vi "OpenPattern.vi"(8 "Error In":errorcluster, 11 "Patten File Path":path caption="path to XML document") -> (0 "Error Out":errorcluster, 3 "Pattern":T1)   [LabVIEW 2012, in "Virtual-PGA.lvlib"]
doc: "This VI loads a pattern from a XML file. The \"Select Pattern Load File Path\" VI should be used to select the XML file."
uses:
  Virtual-PGA.lvlib
  Controls/Pattern.ctl
  Controls/Input.ctl
  <vilib>/xml/Load XML File.vi
  <vilib>/xml/Close Reference(Node).vi
  <vilib>/xml/NI_XML.lvlib
  <resource>/objmgr/DOMUserDefRef.rc
panel:
  out "parse errors":string
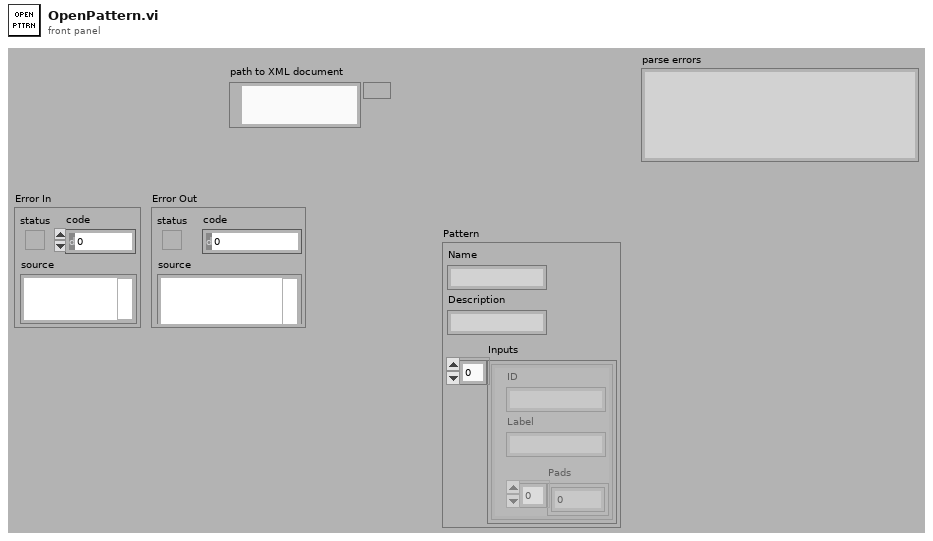
[diagram p1: front panel]
types:
  T1 = typedef "Virtual-PGA.lvlib/Pattern.ctl" = cluster{"Name":string, "Description":string, "Inputs":T2[]}
  T2 = typedef "Virtual-PGA.lvlib/Input.ctl" = cluster{"ID":string, "Label":string, "Pads":u32[]}
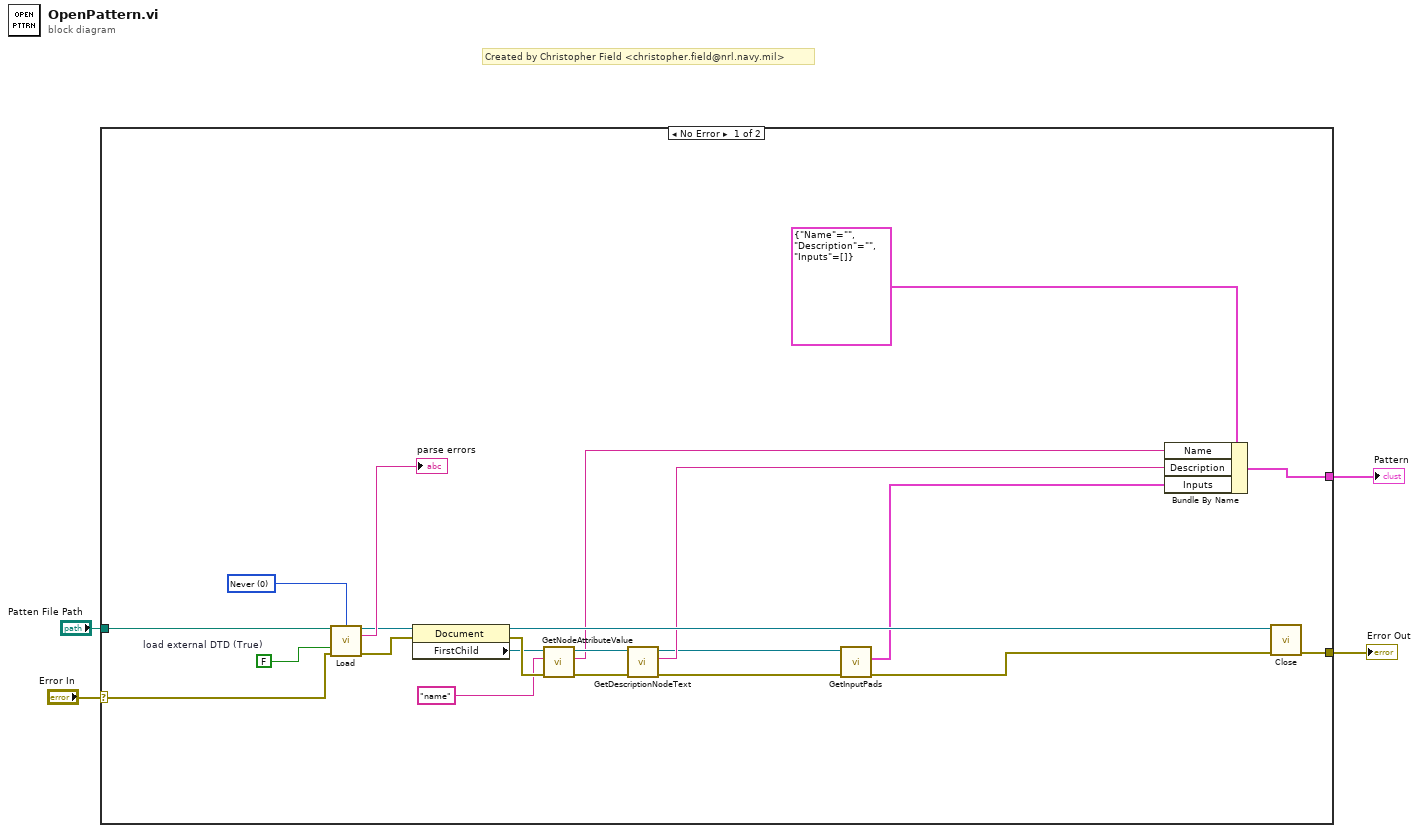
[diagram p0: block diagram]
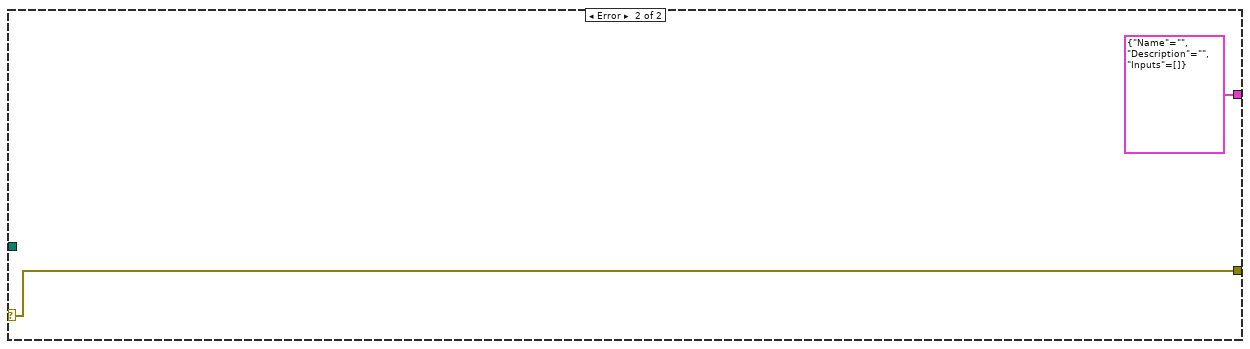
[diagram p2: hidden frame]
diagram:
  # "Created by Christopher Field <christopher.field@nrl.navy.mil>"
  n1 = case shown="No Error" "Error In" {
    selector: "Error In" -> [w8 w27]
    tunnel: "Patten File Path" -> [w26 _]
    tunnel: [w22 w27] -> w3
    tunnel: [w9 T1 {"Name"="", "Description"="", "Inputs"=[]} ("Pattern")] -> w2
    frame No Error {
      w24 = 0 items=["Never", "Always", "Auto"] ("validate on load (Auto)")
      w25 = FALSE  # load external DTD (True)
      n2 = call-poly <vilib>:"Load.vi"("path to XML document"=w26, "validate on load (Auto)"=w24, "load external DTD (True)"=w25, "error in (no error)"=w8) -> ("DOM document out"=w21:refnum<k20>, "parse errors"=→"parse errors":string, "error out"=w19:errorcluster)  [unwired: 9 in]
      n3 = property class="Document"(reference=w21, error in=w19) -> (reference out=w20:refnum<k20>, error out=w18:errorcluster, "FirstChild"=w16:refnum<k20>)
      n4 = call "GetNodeAttributeValue.vi"("Error In"=w18, "Attribute Name"="name", "Node In"=w16) -> ("Error Out"=w15:errorcluster, "Value"=w13:string, "Node Out"=w14:refnum<k20>)  [unwired: 6 in]
      n5 = call "GetDescriptionNodeText.vi"("Error In"=w15, "Pattern Node In"=w14) -> ("Error Out"=w6:errorcluster, "Description"=w12:string, "Pattern Node Out"=w7:refnum<k20>)  [unwired: 7 in]
      n6 = call "GetInputPads.vi"("Error In"=w6, "Pattern Node In"=w7) -> ("Error Out"=w10:errorcluster, "Inputs"=w5:T2[])  [unwired: 7 in, 1 out]
      n7 = Bundle By Name(cluster=T1 {"Name"="", "Description"="", "Inputs"=[]} ("Pattern"), "Name"=w13, "Description"=w12, "Inputs"=w5) -> (w9:T1)
      n8 = call-poly <vilib>:"Close.vi"("error in (no error)"=w10, "node"=w20) -> ("error out"=w22:errorcluster)  [unwired: 7 in]
    }
    frame Error {
    }
  }
  "Error Out" <- w3
  "Pattern" <- w2
